vi "Read.vi"(11 "Local Data Value in":refnum<class "LV Dbl Data Value.lvclass">) -> (2 "Data":T1)   [LabVIEW 2020, in "VolatusHistorian.lvlib" / "LV Dbl Data Value.lvclass"]
uses:
  LV Dbl Data Value.lvclass
  History Data (LV Dbl).ctl
  Channel History (LV Dbl).ctl
  LV Dbl Data Value.lvclass/LV Dbl Data Value.ctl
  VolatusHistorian.lvlib
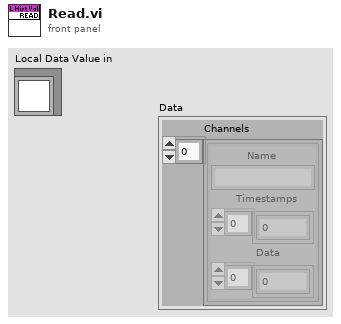
[diagram p1: front panel]
types:
  T1 = typedef "VolatusHistorian.lvlib/History Data (LV Dbl).ctl" = cluster{"Channels":T2[]}
  T2 = typedef "VolatusHistorian.lvlib/Channel History (LV Dbl).ctl" = cluster{"Name":string, "Timestamps":dbl[], "Data":dbl[]}
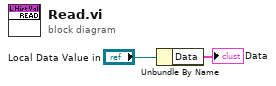
[diagram p0: block diagram]
diagram:
  n1 = Unbundle By Name("Local Data Value in") -> ("Data"=→"Data":T1)
